vi "Cache Response.vi"(7 "ID":string, 8 "error in (no error)":errorcluster, 10 "Response In":refnum<class "Response.lvclass">, 11 "Caching in":refnum<class "Caching.lvclass">) -> (0 "error out":errorcluster, 2 "Response":refnum<class "Response.lvclass">)   [LabVIEW 2020, in "HTTP Server.lvlib" / "Caching.lvclass"]
uses:
  Caching.lvclass
  <vilib>/IlluminatedG/IG HTTP Utils/HTTP Utils/Response/Response.lvclass
  <vilib>/IlluminatedG/IG HTTP Utils/HTTP Utils/File Response/File Response.lvclass
  Caching.lvclass/Caching.ctl
  <vilib>/Utility/miscctls.llb/LVMapReplaceAction.ctl
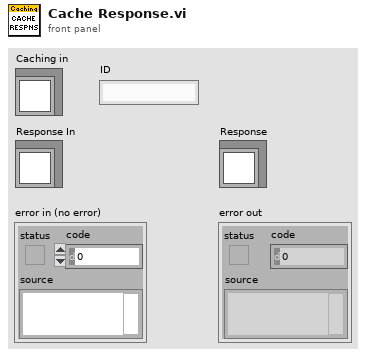
[diagram p1: front panel]
types:
  T1 = typedef "LVMapReplaceAction.ctl" = enum32{"Modify Entry only if found", "Add or Modify Entry", "Delete Entry"}
  T2 = typedef "HTTP Server.lvlib/Caching.lvclass/Memory Cache.ctl" = cluster{"Size":i64, "Map":map{string, T3}}
  T3 = typedef "HTTP Server.lvlib/Caching.lvclass/Cache Item.ctl" = cluster{"ID":string, "File":bool, "Path":path, "Value":string, "Created":timestamp, "Expires":timestamp}
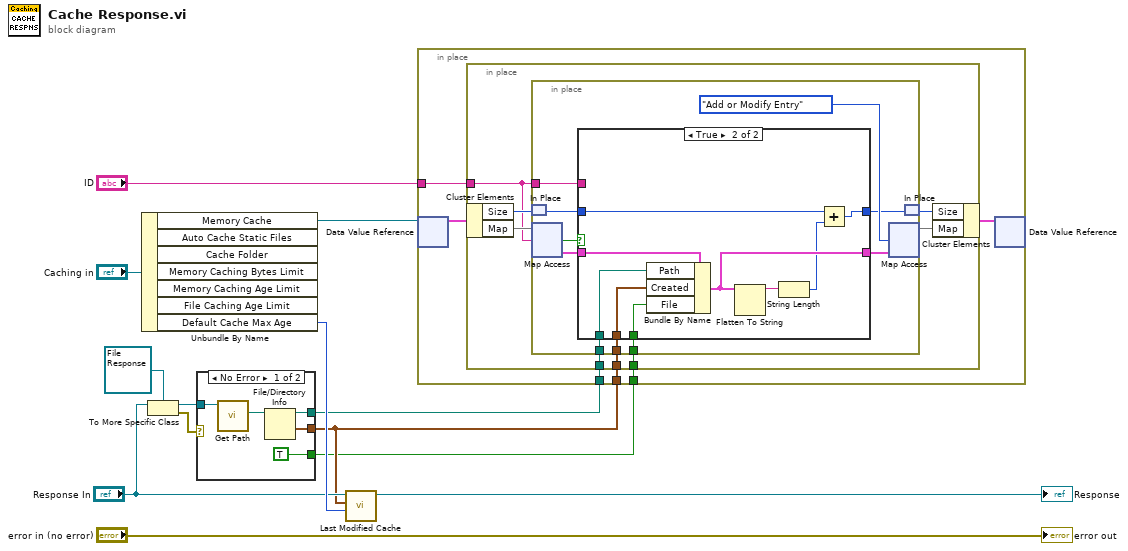
[diagram p0: block diagram]
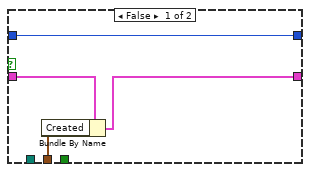
[diagram p2: hidden frame]
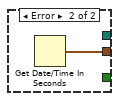
[diagram p3: hidden frame]
diagram:
  n1 = Unbundle By Name("Caching in") -> ("Memory Cache"=w6:refnum<data-value>, "Default Cache Max Age"=w11:i32)  [unwired: 5 out]
  n2 = To More Specific Class(target class=refnum<class "File Response.lvclass"> refnum ("HTTP Utils.lvlib:File Response.lvclass"), reference="Response In") -> (specific class reference=w8:refnum<class "File Response.lvclass">, error out=w9:errorcluster)  [unwired: 1 in]
  n3 = case shown="No Error" w9 {
    tunnel: w8 -> [w18 _]
    tunnel: [w16 w19] -> w4
    tunnel: [w15 _] -> w3
    tunnel: [TRUE _] -> w2
    frame No Error {
      n4 = call <vilib>:"Get Path.vi"("File Response in"=w18) -> ("Path"=w17:path)  [unwired: 8 in, 2 out]
      n5 = File/Directory Info(path=w17) -> (path out=w15:path, last mod=w16:timestamp)  [unwired: 1 in, 5 out]
    }
    frame Error {
      n6 = Get Date/Time In Seconds() -> (seconds since 1Jan1904=w19:timestamp)
    }
  }
  n7 = call <vilib>:"Last Modified Cache.vi"("Max Age"=w11, "Last Modified"=w4, "Response in"="Response In") -> ("Response out"=→"Response":refnum<class "Response.lvclass">)  [unwired: 7 in, 1 out]
  n8 = in-place {
    in-place-border: "ID" -> [w24]
    in-place-border: w4 -> [w23]
    in-place-border: w3 -> [w22]
    in-place-border: w2 -> [w21]
    n9 = in-place-dvr #1(w6) -> (w25:T2)  [unwired: 1 out]
    n10 = in-place {
      in-place-border: w24 -> [w29]
      in-place-border: w23 -> [w30]
      in-place-border: w22 -> [w28]
      in-place-border: w21 -> [w27]
      n11 = in-place-cluster #2(w25) -> ("Size"=w33:i64, "Map"=w31:map{string, T3})
      n12 = in-place {
        in-place-border: w30 -> [w39]
        in-place-border: w29 -> [w37]
        in-place-border: w28 -> [w35]
        in-place-border: w27 -> [w34]
        n13 = in-place-match #3(w33) -> (w41:i64)
        n14 = in-place-map #4(w31, w29) -> (w40:T3, w42:bool)  [unwired: 1 in]
        n15 = case shown="True" w42 {
          tunnel: w41 -> [w45 w50]
          tunnel: w40 -> [w47 w56]
          tunnel: w39 -> [w46 w55]
          tunnel: [w45 w48] -> w38
          tunnel: w37 -> [_ _]
          tunnel: [w44 w52] -> w36
          tunnel: w35 -> [_ w54]
          tunnel: w34 -> [_ w53]
          frame False {
            n16 = Bundle By Name(cluster=w47, "Created"=w46) -> (w44:T3)
          }
          frame True {
            n17 = Bundle By Name(cluster=w56, "Path"=w54, "Created"=w55, "File"=w53) -> (w52:T3)
            n18 = Flatten To String(anything=w52) -> (data string=w51:string)  [unwired: 3 in, 2 out]
            n19 = String Length(string=w51) -> (length=w49:i32)
            n20 = Add(x=w50, y=w49) -> (x+y=w48:i64)
          }
        }
        n21 = in-place-map #4(w36, LVMapReplaceAction."Add or Modify Entry" ("action")) -> (w26:map{string, T3})  [unwired: 2 out]
        n22 = in-place-match #3(w38) -> (w32:i64)
      }
      n23 = in-place-cluster #2("Size"=w32, "Map"=w26) -> (w20:T2)
    }
    n24 = in-place-dvr #1(w20) -> ()  [unwired: 2 out]
  }
  "error out" <- "error in (no error)"
